vi "RawFile Save.vi"(8 "error in (no error)":errorcluster, 9 "File Path (empty)":path, 11 "VI Path (empty)":path) -> (0 "error out":errorcluster)   [LabVIEW 2011]
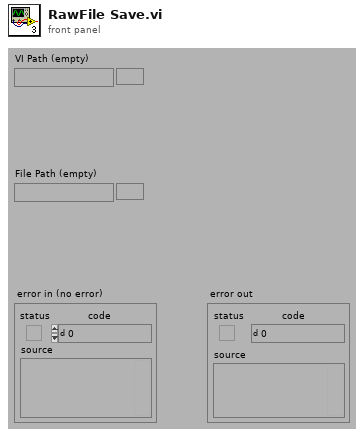
[diagram p1: front panel]
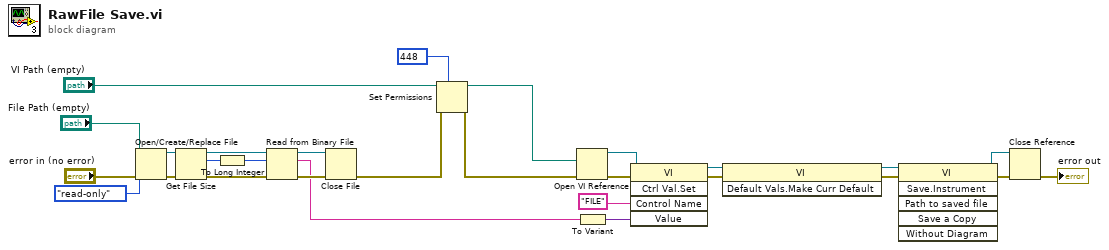
[diagram p0: block diagram]
diagram:
  n1 = Open/Create/Replace File(file path (use dialog)="File Path (empty)", error in="error in (no error)", access (0:read/write)=enum16{"read/write", "read-only", "write-only"}."read-only") -> (refnum out=w11:refnum<file>, error out=w13:errorcluster)  [unwired: 4 out]
  n2 = Get File Size(file=w11, error in=w13) -> (refnum out=w10:refnum<file>, size (in bytes)=w9:i64, 0:w12:errorcluster)
  n3 = To Long Integer(number=w9) -> (32bit integer=w8:i32)
  n4 = Read from Binary File(8:w12, 10:w8, 11:w10) -> (0:w16:errorcluster, 2:w15:string, 3:w14:refnum<file>)  [unwired: 4 out]
  n5 = Close File(refnum=w14, error in=w16) -> (error out=w3:errorcluster)  [unwired: 1 out]
  n6 = Set Permissions(7:i16 448 ("permissions"), 8:w3, 11:"VI Path (empty)") -> (0:w2:errorcluster, 3:w4:path)  [unwired: 2 out]
  n7 = Open VI Reference(vi path=w4, error in (no error)=w2) -> (vi reference=w27:refnum<vi>, error out=w28:errorcluster)  [unwired: 4 out]
  n8 = To Variant(anything=w15) -> (Variant=w26:variant)
  n9 = invoke class="VI" method="Ctrl Val.Set"(reference=w27, error in=w28, "Control Name"="FILE", "Value"=w26) -> (reference out=w24:refnum<vi>, error out=w25:errorcluster)  [unwired: 1 in, 3 out]
  n10 = invoke class="VI" method="Default Vals.Make Curr Default"(reference=w24, error in=w25) -> (reference out=w22:refnum<vi>, error out=w23:errorcluster)  [unwired: 1 in, 1 out]
  n11 = invoke class="VI" method="Save.Instrument"(reference=w22, error in=w23) -> (reference out=w20:refnum<vi>, error out=w21:errorcluster)  [unwired: 4 in, 4 out]
  n12 = Close Reference(reference=w20, error in (no error)=w21) -> (error out=→"error out":errorcluster)
